vi "Resistance_test.vi"() -> ()   [LabVIEW 2017]
uses:
  <vilib>/DAQmx/write.llb/DAQmx Write (Analog DBL 1Chan 1Samp).vi
  <vilib>/DAQmx/create/channels.llb/DAQmx Create Channel (AI-Voltage-Basic).vi
  <vilib>/DAQmx/create/channels.llb/DAQmx Create Channel (AO-Voltage-Basic).vi
  <vilib>/DAQmx/miscellaneous.llb/DAQmx Fill In Error Info.vi
panel:
  out "Voltage Sum":dbl
  out "SpectrumGraph":cluster{i32[], dbl[]}(graph)
  in  "Rsh, Ohm":dbl=5091.0 min=0.0
  out "Voltage Output.Min":dbl
  out "Voltage Output.Max":dbl=2.0
  out "U.Min":dbl=-0.1
  out "U.Max":dbl=0.1
  out "Ush.Min":dbl=-2.0
  out "Ush.Max":dbl=2.0
  out "size(s)":i32=100
  out "Average Resistance, Ohm":dbl=98.20735292590594
  in  "Averaging points":i32=100
  in  "DAQ channel In Voltage Output":tag="DAQ6363/ao0"
  out "Resistance, Ohm":dbl=98.23321199097627 min=-6000.0 max=6000.0 format="%#.2f"
  out "Current, mA":dbl=0.3847962107212662 min=-6000.0 max=6000.0 format="%#.5f"
  in  "Voltage Output, V":dbl=2.0 min=0.0 max=10.0 format="%#.2f"
  out "error out":errorcluster
  in  "stop":bool
  in  "Error In (no error)":errorcluster
  out "Voltage Ush, V":dbl=1.9589975087819662 min=-6000.0 max=6000.0 format="%#.4f"
  in  "DAQ channel In Voltage U":tag="DAQ6363/ai5"
  in  "DAQ channel In Voltage Ush":tag="DAQ6363/ai4"
  out "Voltage U, V":dbl=0.03779976774110652 min=-6000.0 max=6000.0 format="%#.4f"
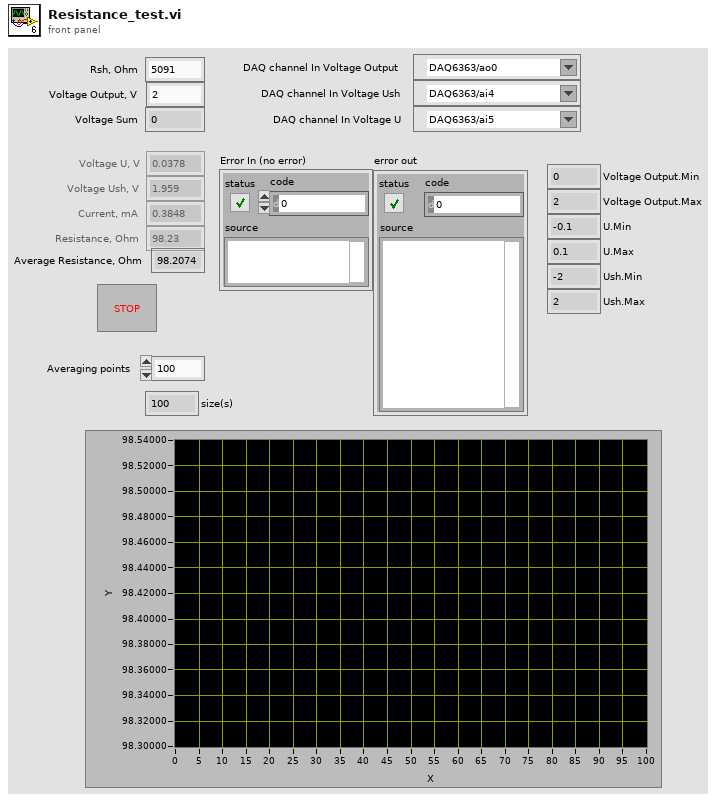
[diagram p1: front panel]
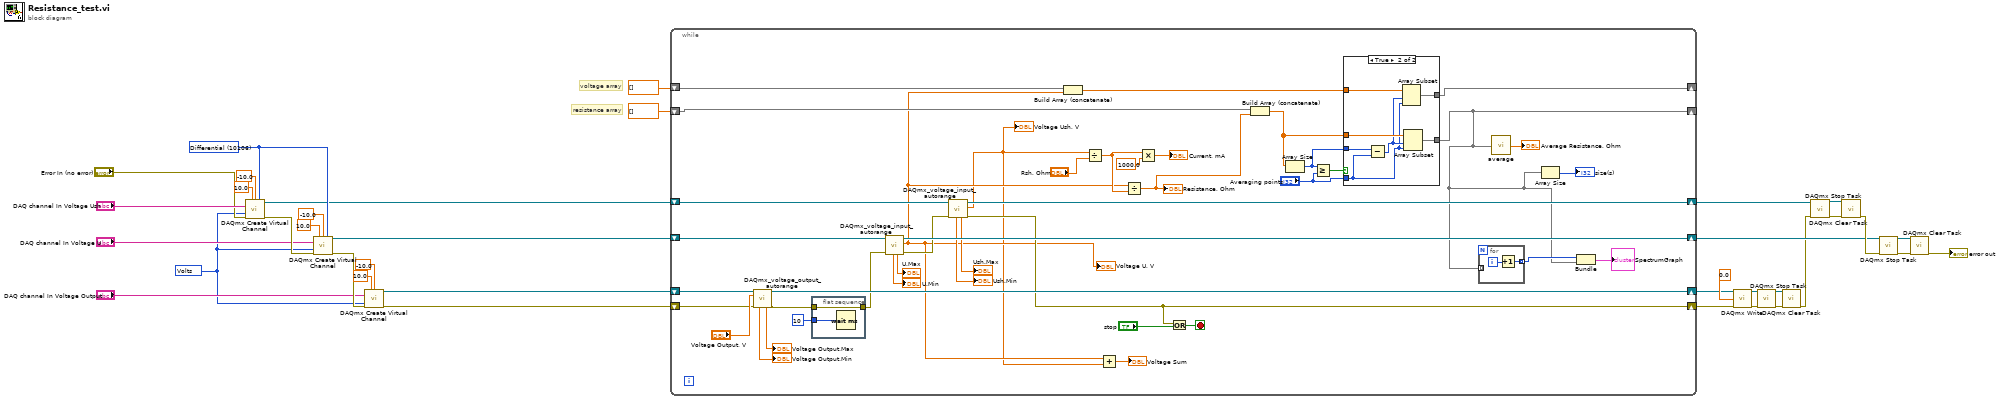
[diagram p0: block diagram]
diagram:
  w13 = 10106 items=["Default"=-1, "RSE"=10083, "NRSE"=10078, "Differential"=10106, "Pseudodifferential"=12529] ("input terminal configuration")
  w14 = 10348 items=["Volts"=10348, "From Custom Scale"=10065] ("units")
  # "resistance array"
  # "voltage array"
  n1 = call-poly <vilib>:"DAQmx Create Virtual Channel.vi"("maximum value"=10.0, "minimum value"=-10.0, "input terminal configuration"=w13, "physical channels"="DAQ channel In Voltage Ush", "units"=w14, "error in"="Error In (no error)") -> ("task out"=w5:refnum<k21>, "error out"=w36:errorcluster)  [unwired: 8 in]
  n2 = call-poly <vilib>:"DAQmx Create Virtual Channel.vi"("maximum value"=10.0, "minimum value"=-10.0, "input terminal configuration"=w13, "physical channels"="DAQ channel In Voltage U", "units"=w14, "error in"=w36) -> ("task out"=w6:refnum<k21>, "error out"=w24:errorcluster)  [unwired: 8 in]
  n3 = call-poly <vilib>:"DAQmx Create Virtual Channel.vi"("maximum value"=10.0, "minimum value"=-10.0, "physical channels"="DAQ channel In Voltage Output", "units"=w14, "error in"=w24) -> ("task out"=w8:refnum<k21>, "error out"=w7:errorcluster)  [unwired: 9 in]
  n4 = while {
    shift-right: [w55] -> w27
    shift-left: w5 -> [w57]
    shift-right: [w60] -> w26
    shift-left: w6 -> [w62]
    shift-right: [w54] -> w16
    shift-left: w7 -> [w64]
    shift-right: [w37] -> _
    shift-left: dbl[] [] -> [w76]
    shift-right: [w68] -> w2
    shift-left: w8 -> [w69]
    shift-right: [w38] -> _
    shift-left: dbl[] [] -> [w50]
    stop <- w77 stop-if-true
    n5 = call "DAQmx_voltage_output_autorange.vi"("DAQ task Voltage Output in"=w69, "Voltage Output, V"="Voltage Output, V", "error in (no error)"=w64) -> ("DAQ task Voltage Output out"=w68:refnum<k21>, "AO.Min"=→"Voltage Output.Min":dbl, "AO.Max"=→"Voltage Output.Max":dbl, "error out"=w63:errorcluster)  [unwired: 9 in]
    n6 = flat-sequence {
      tunnel: [w91] -> w61
      tunnel: w63 -> [w91]
      tunnel: u32 10 ("milliseconds to wait") -> [w90]
      frame #0 {
        n7 = Wait (ms)(milliseconds to wait=w90) -> ()  [unwired: 1 out]
      }
    }
    n8 = call "DAQmx_voltage_input_autorange.vi"("error in (no error)"=w61, "DAQ task Voltage in"=w62) -> ("error out"=w56:errorcluster, "data"=w46:dbl, "task out"=w60:refnum<k21>, "AI.Max"=→"U.Max":dbl, "AI.Min"=→"U.Min":dbl)  [unwired: 5 in]
    "Voltage U, V" <- w46
    n9 = call "DAQmx_voltage_input_autorange.vi"("error in (no error)"=w56, "DAQ task Voltage in"=w57) -> ("error out"=w54:errorcluster, "data"=w45:dbl, "task out"=w55:refnum<k21>, "AI.Max"=→"Ush.Max":dbl, "AI.Min"=→"Ush.Min":dbl)  [unwired: 5 in]
    "Voltage Ush, V" <- w45
    n10 = Build Array (concatenate)(w50, w46) -> (w43:dbl[])
    n11 = Divide(x=w45, y="Rsh, Ohm") -> (x/y=w74:dbl)
    n12 = Add(x=w46, y=w45) -> (x+y=→"Voltage Sum":dbl)
    n13 = Divide(x=w46, y=w74) -> (x/y=w51:dbl)
    "Resistance, Ohm" <- w51
    n14 = Multiply(x=w74, y=1000.0) -> (x*y=→"Current, mA":dbl)
    n15 = Or(x=w54, y="stop") -> (x .or. y?=w77:bool)
    n16 = Build Array (concatenate)(w76, w51) -> (w75:dbl[])
    n17 = Array Size(array=w75) -> (size(s)=w49:i32)
    n18 = Greater Or Equal?(x=w49, y="Averaging points") -> (x >= y?=w48:bool)
    n19 = case shown="True" w48 {
      tunnel: w75 -> [w82 w89]
      tunnel: w49 -> [_ w88]
      tunnel: "Averaging points" -> [_ w84]
      tunnel: [w82 w87] -> w37
      tunnel: w43 -> [w81 w86]
      tunnel: [w81 w83] -> w38
      frame False {
      }
      frame True {
        n20 = Subtract(x=w88, y=w84) -> (x-y=w85:i32)
        n21 = Array Subset(array=w86, index=w85, length=w84) -> (w83:dbl[])
        n22 = Array Subset(array=w89, index=w85, length=w84) -> (w87:dbl[])
      }
    }
    n23 = for {
      tunnel: [w79] -> w41 mode=indexing
      tunnel: w37 -> [_] mode=indexing
      i -> [w80]
      n24 = Increment(x=w80) -> (x+1=w79:i32)
    }
    n25 = call "average.vi"("Array"=w37) -> ("Average"=→"Average Resistance, Ohm":dbl)
    n26 = Array Size(array=w37) -> (size(s)=→"size(s)":i32)
    n27 = Bundle(w41, w37) -> (→"SpectrumGraph":cluster{i32[], dbl[]})  [unwired: 1 in]
  }
  n28 = call-poly <vilib>:"DAQmx Write.vi"("task/channels in"=w2, "data"=0.0, "error in"=w16) -> ("task out"=w20:refnum<k21>, "error out"=w18:errorcluster)  [unwired: 10 in, 1 out]
  n29 = call <vilib>:"DAQmx Stop Task.vi"("task/channels in"=w20, "error in"=w18) -> ("task out"=w22:refnum<k21>, "error out"=w21:errorcluster)  [unwired: 12 in]
  n30 = call <vilib>:"DAQmx Clear Task.vi"("task in"=w22, "error in"=w21) -> ("error out"=w17:errorcluster)  [unwired: 13 in]
  n31 = call <vilib>:"DAQmx Stop Task.vi"("task/channels in"=w27, "error in"=w17) -> ("task out"=w34:refnum<k21>, "error out"=w33:errorcluster)  [unwired: 12 in]
  n32 = call <vilib>:"DAQmx Clear Task.vi"("task in"=w34, "error in"=w33) -> ("error out"=w30:errorcluster)  [unwired: 13 in]
  n33 = call <vilib>:"DAQmx Stop Task.vi"("task/channels in"=w26, "error in"=w30) -> ("task out"=w31:refnum<k21>, "error out"=w32:errorcluster)  [unwired: 12 in]
  n34 = call <vilib>:"DAQmx Clear Task.vi"("task in"=w31, "error in"=w32) -> ("error out"=→"error out":errorcluster)  [unwired: 13 in]
